vi "Set Device.vi"(8 "error in (no error)":errorcluster, 10 "Device":refnum<class "Device.lvclass">, 11 "DeviceDetailPanel in":refnum<class "DeviceDetailPanel.lvclass">) -> (0 "error out":errorcluster, 3 "DeviceDetailPanel out":refnum<class "DeviceDetailPanel.lvclass">)   [LabVIEW 2020, in "PicoG-App.lvlib" / "DeviceDetailPanel.lvclass"]
uses:
  DeviceDetailPanel.lvclass
  Device/Device.lvclass
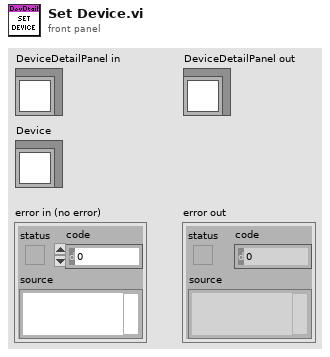
[diagram p1: front panel]
types:
  T1 = typedef "PicoG-App.lvlib/DeviceDetailPanel.lvclass/Ref Data.ctl" = cluster{"Device":refnum<class "Device.lvclass">}
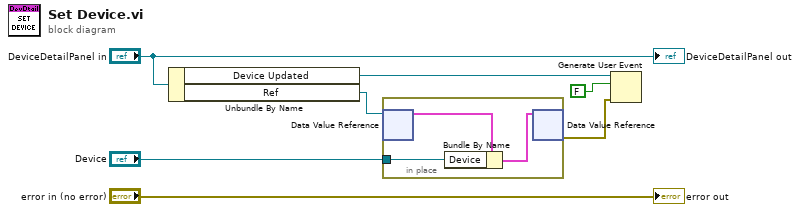
[diagram p0: block diagram]
diagram:
  n1 = Unbundle By Name("DeviceDetailPanel in") -> ("Device Updated"=w3:refnum<user-event>, "Ref"=w6:refnum<data-value>)
  n2 = in-place {
    in-place-border: "Device" -> [w8]
    n3 = in-place-dvr #1(w6) -> (w10:T1)  [unwired: 1 out]
    n4 = Bundle By Name(cluster=w10, "Device"=w8) -> (w9:T1)
    n5 = in-place-dvr #1(w9) -> (w1:errorcluster)  [unwired: 1 out]
  }
  n6 = Generate User Event(user event=w3, event data cluster=FALSE ("event data"), error in=w1) -> ()  [unwired: 1 in, 2 out]
  "error out" <- "error in (no error)"
  "DeviceDetailPanel out" <- "DeviceDetailPanel in"
